vi "Test1.vi"() -> ()   [LabVIEW 2014]
uses:
  controls/Data1.ctl
  controls/ReadScan1States.ctl
panel:
  in  "Read":bool
  out "Data":T1
  out "Coils":bool[](array[boolean])
  in  "stop":bool
  out "error out":errorcluster
  in  "error in (no error)":errorcluster
  # "SENSOR1"
  # "SENSOR2"
  # "SENSOR3"
  # "日期"
  # "機種名稱"
  # "機種代號"
  # "商品條碼"
  # "OK"
  # "台"
  # "NG"
  # "台"
  # "總計"
  # "台"
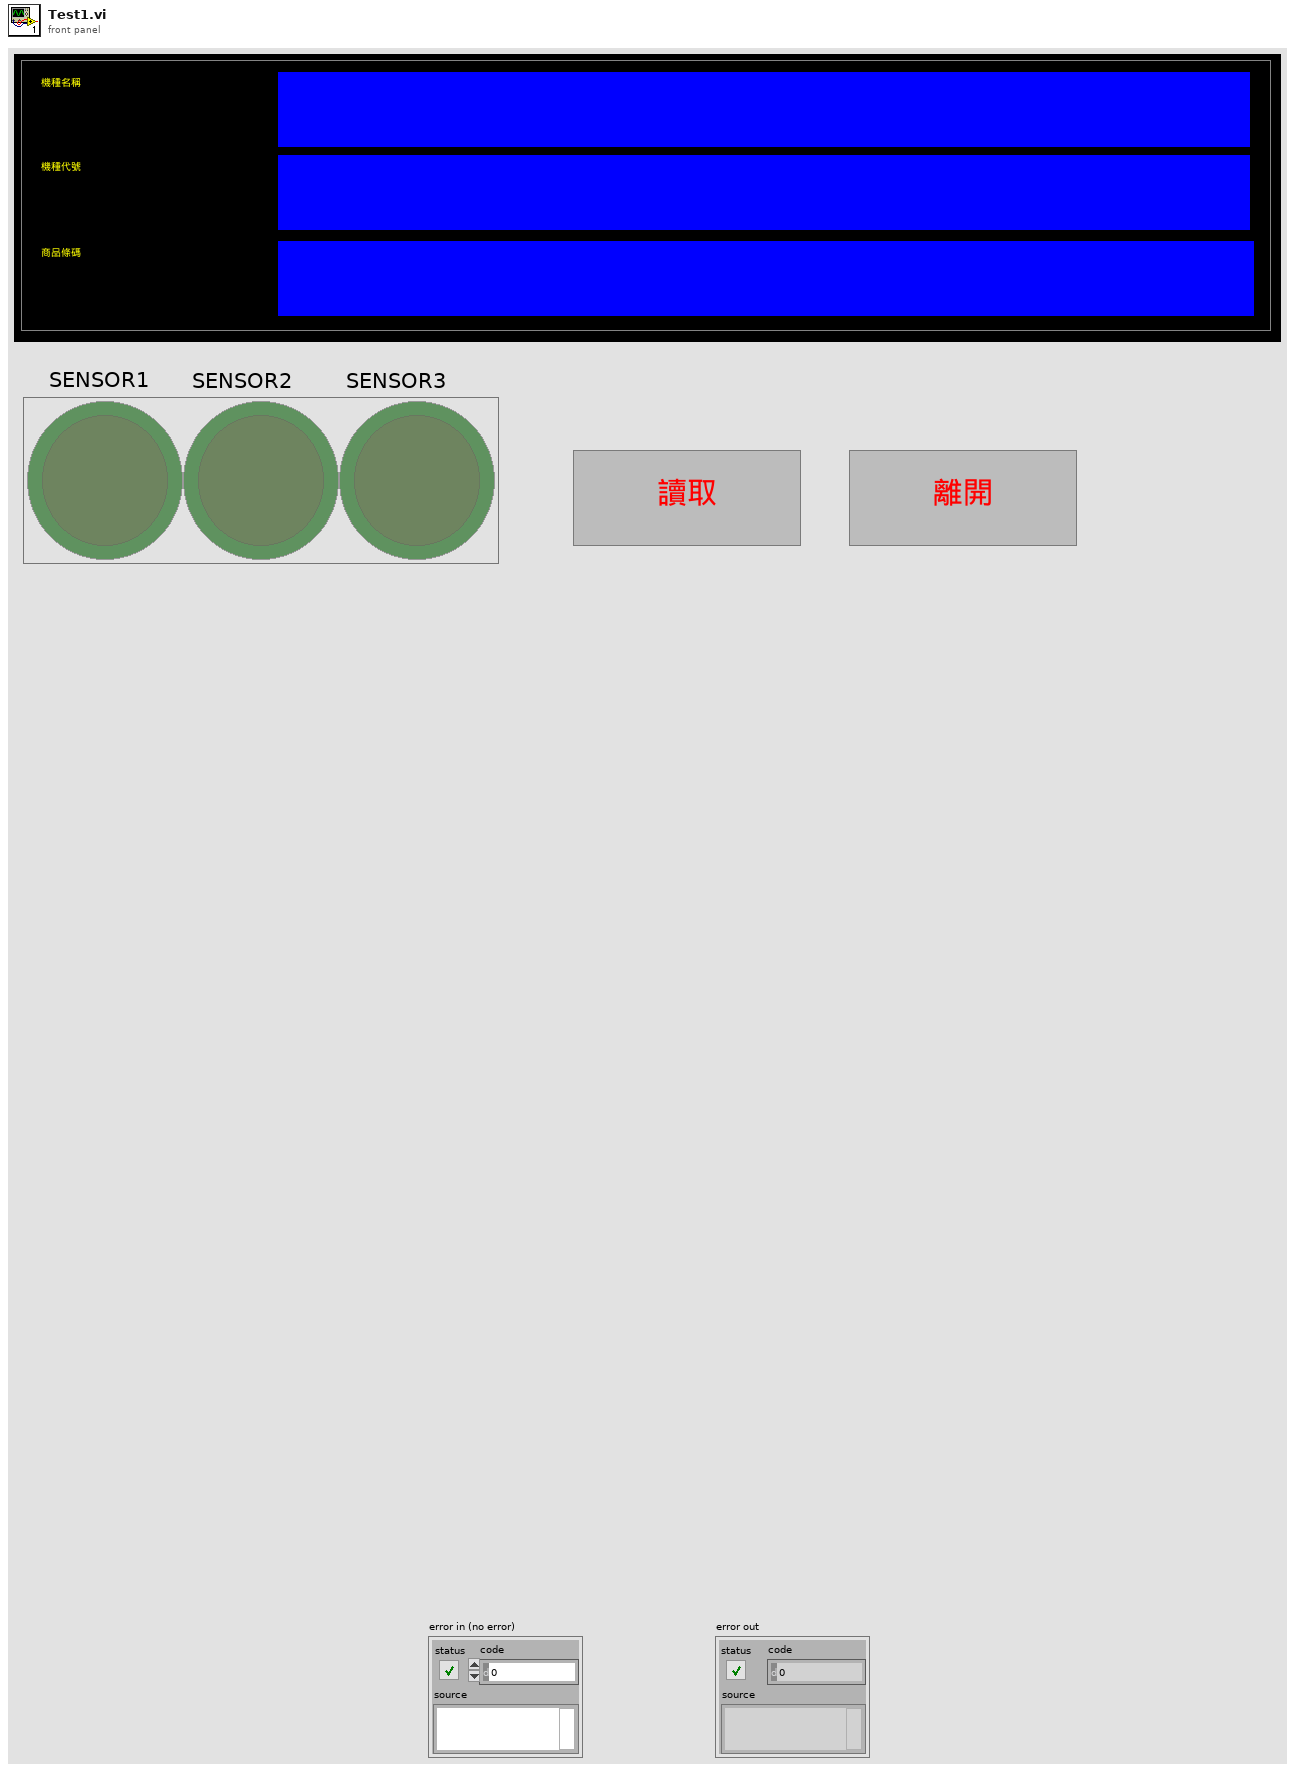
[diagram p1: front panel]
types:
  T1 = typedef "Data1.ctl" = cluster{"Date":string, "BarCode1":string, "BarCode2":string, "BarCode3":string, "Message":string, "OK Count":u16, "NG Count":u16, "Total Count":u16, "ModelData":string[][], "OK&NG":bool, "COM1":refnum<visa-resource-name>, "COM2":refnum<visa-resource-name>, "IO":i32, "Time":u32, "TCP":refnum<k5>, "TCP 2":refnum<k5>}
  T2 = typedef "ReadScan1States.ctl" = enum16{"Initialize", "Init2", "Step1", "Step2", "Step3", "Step4", "One", "Two", "Three", "Four", "Five", "End", "Stop"}
  T3 = typedef "Data.ctl" = cluster{"Date":string, "BarCode1":string, "BarCode2":string, "BarCode3":string, "Message":string, "OK Count":u16, "NG Count":u16, "Total Count":u16, "ModelData":string[][], "OK&NG":bool, "COM1":refnum<visa-resource-name>, "COM2":refnum<visa-resource-name>, "IO":i32, "Time":u32, "TCP":refnum<k5>, "TCP 2":refnum<k5>}
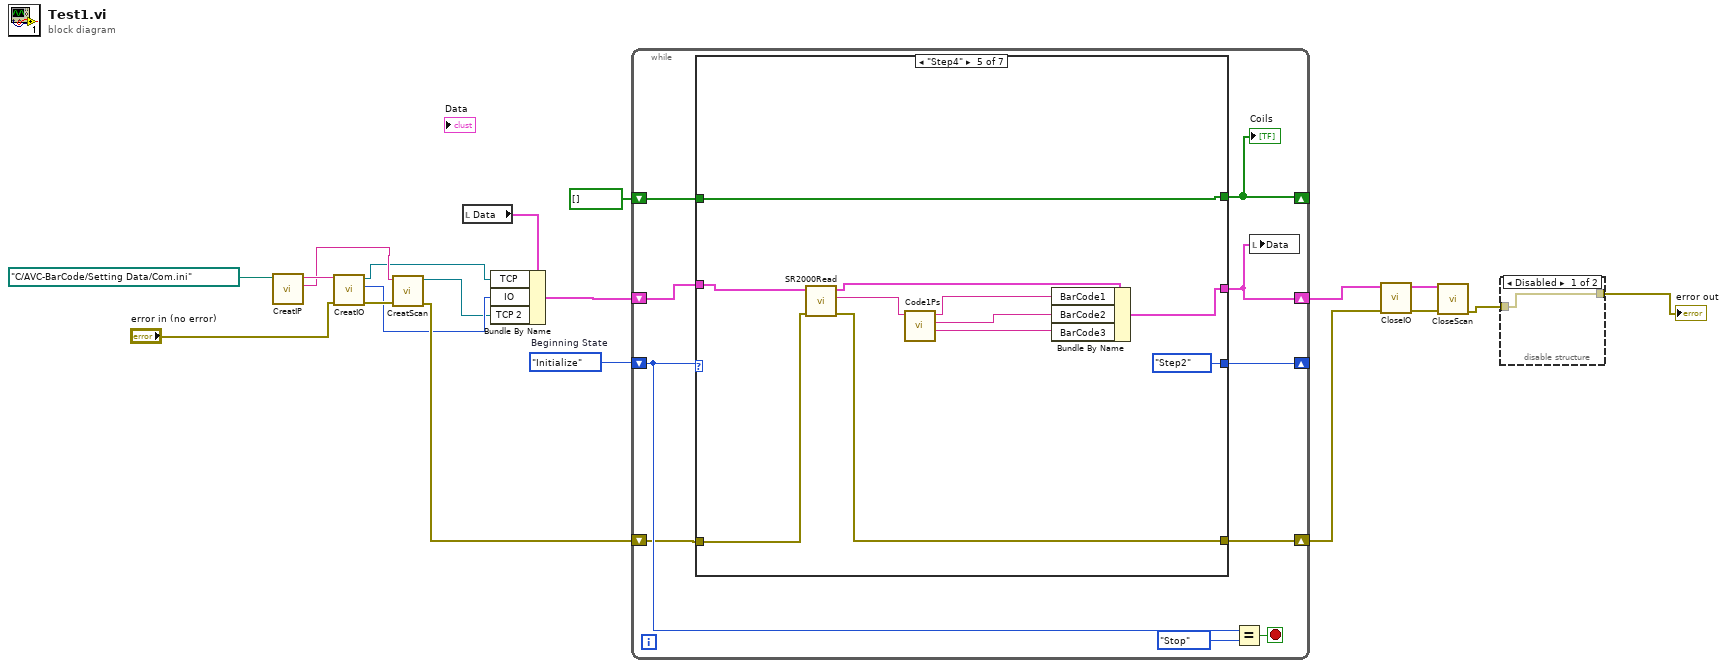
[diagram p0: block diagram]
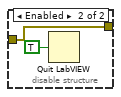
[diagram p2: hidden frame]
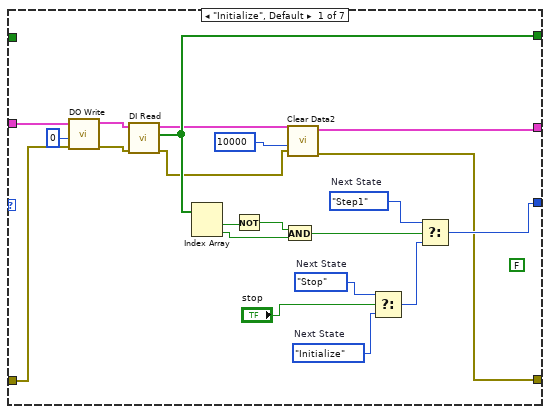
[diagram p3: hidden frame]
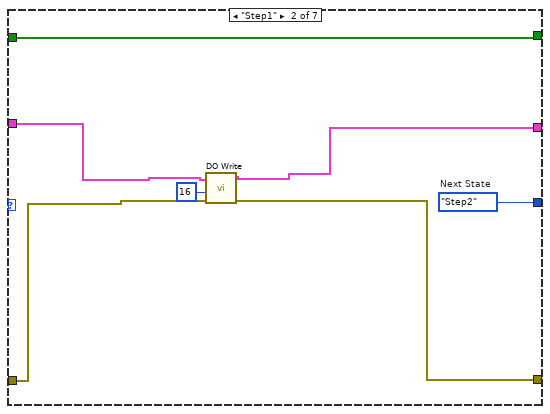
[diagram p4: hidden frame]
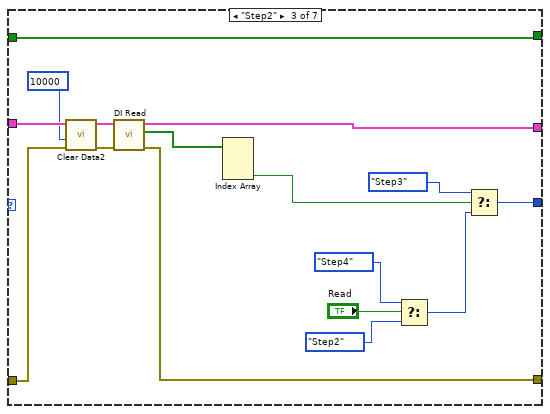
[diagram p5: hidden frame]
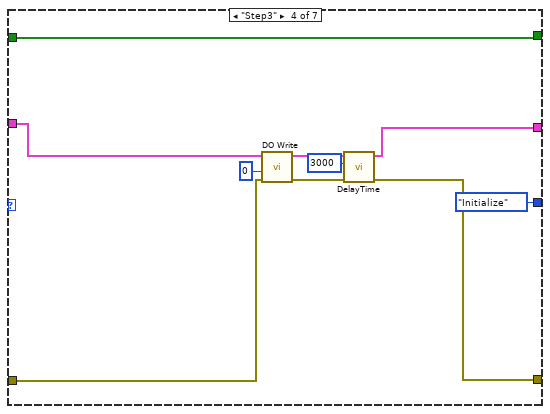
[diagram p6: hidden frame]
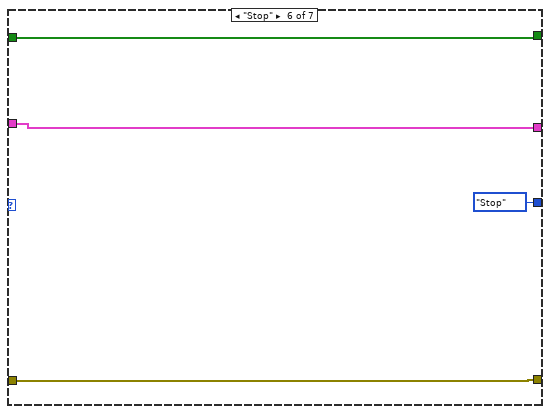
[diagram p7: hidden frame]
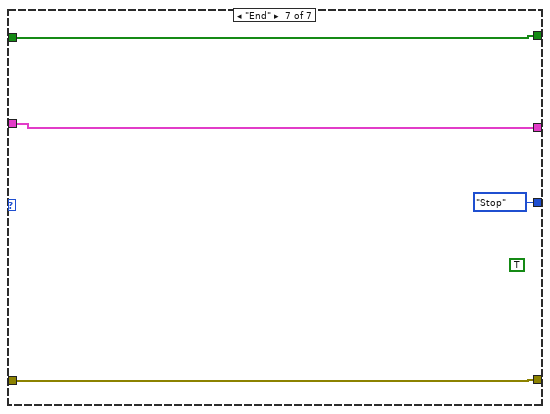
[diagram p8: hidden frame]
diagram:
  w19 = ReadScan1States."Initialize"  # Beginning State
  n1 = call "CreatIP.vi"("file Path"=path "C:/AVC-BarCode/Setting Data/Com.ini" ("IO Path")) -> ("Scan IP"=w10:string, "IO IP"=w11:string)  [unwired: 9 in]
  n2 = call "CreatIO.vi"("error in (no error)"="error in (no error)", "address"=w11) -> ("error out"=w8:errorcluster, "IO"=w5:i32, "TCP Out"=w7:refnum<k5>)  [unwired: 7 in]
  n3 = call "CreatScan.vi"("error in (no error)"=w8, "address"=w10) -> ("error out"=w6:errorcluster, "TCP Out"=w4:refnum<k5>)  [unwired: 7 in, 1 out]
  n4 = local read "Data"() -> (w12:T1)
  n5 = Bundle By Name(cluster=w12, "TCP"=w7, "IO"=w5, "TCP 2"=w4) -> (w17:T1)
  n6 = while {
    shift-right: [w26] -> _
    shift-left: w19 -> [w27]
    shift-right: [w20] -> w16
    shift-left: w17 -> [w24]
    shift-right: [w23] -> w15
    shift-left: w6 -> [w25]
    shift-right: [w21] -> _
    shift-left: bool[] [] ("Coils") -> [w22]
    stop <- w29 stop-if-true
    n7 = case shown="\"Step4\"" w27 {
      tunnel: [w49 w54 w71 ReadScan1States."Initialize" ("Next State") ReadScan1States."Step2" ("Next State") ReadScan1States."Stop" ("Next State") ReadScan1States."Stop" ("Next State")] -> w26
      tunnel: w25 -> [w37 w55 w66 w80 w90 w96 w100]
      tunnel: w24 -> [w39 w56 w67 w81 w93 w97 w101]
      tunnel: [w32 w52 w58 w77 w91 w97 w101] -> w20
      tunnel: [w30 w53 w72 w75 w89 w96 w100] -> w23
      tunnel: [w40 w51 w68 w79 w94 w95 w99] -> w21
      tunnel: w22 -> [_ w51 w68 w79 w94 w95 w99]
      frame "Initialize", Default {
        w44 = ReadScan1States."Stop"  # Next State
        (unwired) FALSE
        w50 = ReadScan1States."Step1"  # Next State
        w42 = ReadScan1States."Initialize"  # Next State
        n8 = call "DO Write.vi"("error in (no error)"=w37, "data"=u8 0, "Data In"=w39) -> ("error out"=w36:errorcluster, "Data Out"=w38:T3)  [unwired: 7 in]
        n9 = call "DI Read.vi"("error in (no error)"=w36, "Data In"=w38) -> ("error out"=w31:errorcluster, "Coils"=w40:bool[], "Data Out"=w33:T3)  [unwired: 7 in]
        n10 = Index Array(array=w40) -> (element #1=w48:bool, element #2=w46:bool)  [unwired: 2 in]
        n11 = Not(x=w48) -> (.not. x?=w47:bool)
        n12 = And(x=w47, y=w46) -> (x .and. y?=w45:bool)
        n13 = call "Clear Data2.vi"("error in (no error)"=w31, "Time"=u32 10000, "Data In"=w33) -> ("error out"=w30:errorcluster, "Data Out"=w32:T3)  [unwired: 7 in]
        n14 = Select(t=w44, s="stop", f=w42) -> (s? t:f=w41:T2)
        n15 = Select(t=w50, s=w45, f=w41) -> (s? t:f=w49:T2)
      }
      frame "Step1" {
        w54 = ReadScan1States."Step2"  # Next State
        n16 = call "DO Write.vi"("error in (no error)"=w55, "data"=u8 16, "Data In"=w56) -> ("error out"=w53:errorcluster, "Data Out"=w52:T3)  [unwired: 7 in]
      }
      frame "Step2" {
        n17 = call "Clear Data2.vi"("error in (no error)"=w66, "Time"=u32 10000, "Data In"=w67) -> ("error out"=w65:errorcluster, "Data Out"=w64:T3)  [unwired: 7 in]
        n18 = call "DI Read.vi"("error in (no error)"=w65, "Data In"=w64) -> ("error out"=w72:errorcluster, "Coils"=w73:bool[], "Data Out"=w58:T3)  [unwired: 7 in]
        n19 = Index Array(array=w73) -> (element #3=w70:bool)  [unwired: 3 in, 2 out]
        n20 = Select(t=ReadScan1States."Step4", s="Read", f=ReadScan1States."Step2" ("Next State")) -> (s? t:f=w59:T2)
        n21 = Select(t=ReadScan1States."Step3", s=w70, f=w59) -> (s? t:f=w71:T2)
      }
      frame "Step3" {
        n22 = call "DO Write.vi"("error in (no error)"=w80, "data"=u8 0, "Data In"=w81) -> ("error out"=w76:errorcluster, "Data Out"=w78:T3)  [unwired: 7 in]
        n23 = call "DelayTime.vi"("error in (no error)"=w76, "Time"=u32 3000, "Data In"=w78) -> ("error out"=w75:errorcluster, "Data Out"=w77:T3)  [unwired: 7 in]
      }
      frame "Step4" {
        n24 = call "SR2000Read.vi"("error in (no error)"=w90, "Data In"=w93) -> ("error out"=w89:errorcluster, "BarCodeRead"=w88:string, "Data Out"=w92:T3)  [unwired: 7 in]
        n25 = call "Code1Ps.vi"("Code1 In"=w88) -> ("紙箱號碼"=w85:string, "機種代號"=w86:string, "機種名"=w87:string)  [unwired: 8 in]
        n26 = Bundle By Name(cluster=w92, "BarCode1"=w87, "BarCode2"=w86, "BarCode3"=w85) -> (w91:T3)
      }
      frame "Stop" {
      }
      frame "End" {
        (unwired) TRUE
      }
    }
    "Coils" <- w21
    n27 = Equal?(x=w27, y=ReadScan1States."Stop" ("States")) -> (x = y?=w29:bool)
    n28 = local write "Data"(w20) -> ()
  }
  n29 = call "CloseIO.vi"("error in (no error)"=w15, "Data In"=w16) -> ("error out"=w2:errorcluster, "Data Out"=w3:T3)  [unwired: 8 in]
  n30 = call "CloseScan.vi"("error in (no error)"=w2, "Data In"=w3) -> ("error out"=w1:errorcluster)  [unwired: 8 in, 1 out]
  n31 = disable-structure shown="Disabled" {
    disable-tunnel: w1 -> [w103 w104]
    disable-tunnel: [w103 w104] -> w13
    frame Disabled {
    }
    frame Enabled {
      n32 = Quit LabVIEW(quit? (T)=TRUE) -> ()
    }
  }
  "error out" <- w13
